vi "Hatch4barCollisionAvoidance.vi"(10 "Current4barSetpoint":dbl, 11 "Hatch Setpoint":dbl) -> (3 "Modified 4bar setpoint":dbl)   [LabVIEW 2018]
uses:
  Infrastructure/Constants.vi
  Robot Global Data.vi
panel:
  out "On floor":bool
  out "currently in bad zone":bool
  out "INtending to move throug floor":bool
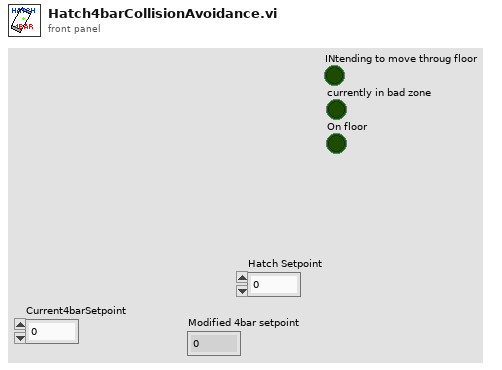
[diagram p1: front panel]
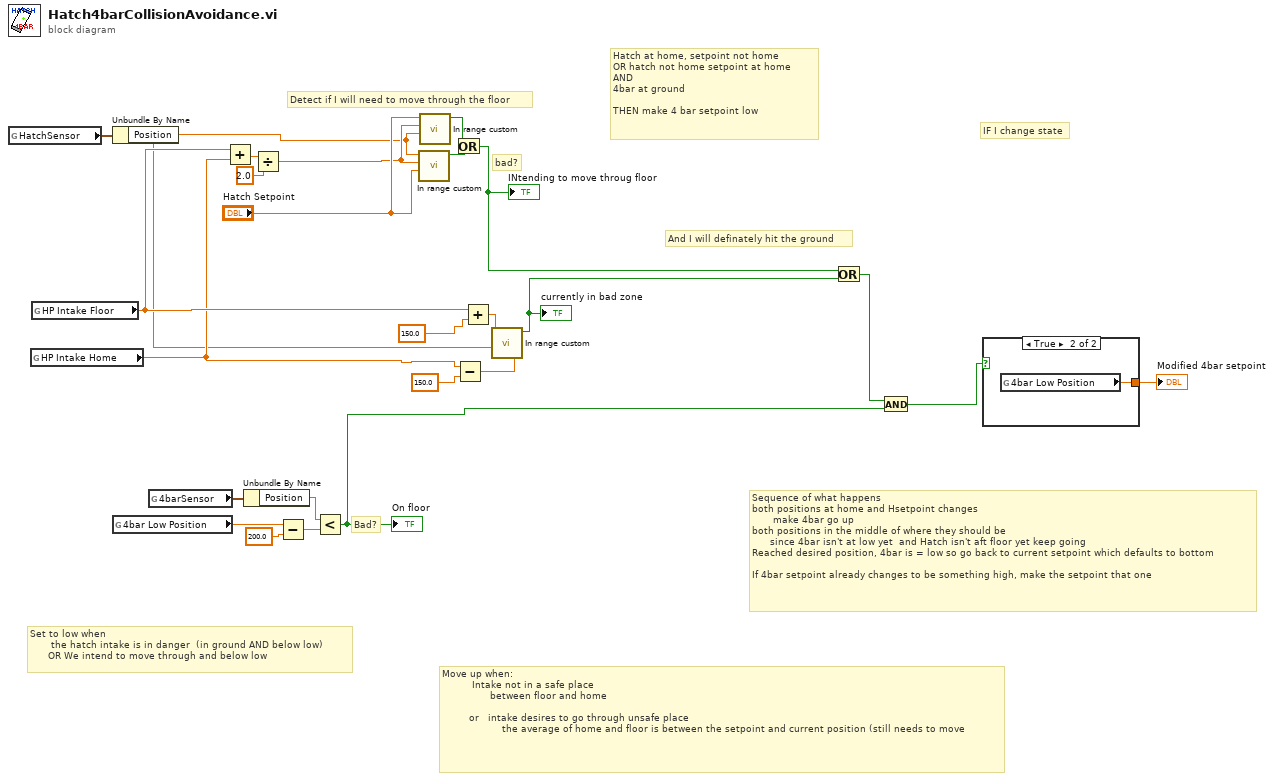
[diagram p0: block diagram]
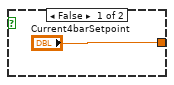
[diagram p2: hidden frame]
diagram:
  # "Set to low when \n       the hatch intake is in danger  (in ground AND below low)\n      OR We intend to move through and below low"
  # "Move up when: \n          Intake not in a safe place\n                between floor and home\n\n         or   intake desires to go through unsafe place\n                    the average of home and floor is between the setpoint and current position (still needs to move"
  # "bad?"
  # "Bad?"
  # "Detect if I will need to move through the floor"
  # "And I will definately hit the ground"
  # "IF I change state"
  # "Sequence of what happens\nboth positions at home and Hsetpoint changes\n       make 4bar go up\nboth positions in the middle of where they should be\n      since 4bar isn't at low yet  and Hatch isn't aft floor yet keep going\nReached desired position, 4bar is = low so go back to current setpoint which defaults to bottom\n\nIf 4bar setpoint already changes to be something high, make the setpoint that one"
  # "Hatch at home, setpoint not home\nOR hatch not home setpoint at home \nAND\n4bar at ground\n\nTHEN make 4 bar setpoint low"
  n1 = global read "Robot Global Data.vi" "HatchSensor"() -> (w25:cluster{"Position":dbl, "Velocity":dbl})
  n2 = global read "Constants.vi" "HP Intake Home"() -> (w10:dbl)
  n3 = global read "Constants.vi" "HP Intake Floor"() -> (w11:dbl)
  n4 = Unbundle By Name(w25) -> ("Position"=w1:dbl)
  n5 = global read "Constants.vi" "4bar Low Position"() -> (w14:dbl)
  n6 = global read "Robot Global Data.vi" "4barSensor"() -> (w24:cluster{"Position":dbl, "Velocity":dbl})
  n7 = Add(x=w11, y=w10) -> (x+y=w21:dbl)
  n8 = Unbundle By Name(w24) -> ("Position"=w22:dbl)
  n9 = Divide(x=w21, y=2.0) -> (x/y=w2:dbl)
  n10 = Subtract(x=w14, y=200.0 ("x")) -> (x-y=w15:dbl)
  n11 = Less?(x=w22, y=w15) -> (x < y?=w17:bool)
  "On floor" <- w17
  n12 = call "In range custom.vi"("Lower limit"="Hatch Setpoint", "x"=w2, "Upper limit"=w1) -> ("In range?"=w5:bool)  [unwired: 8 in]
  n13 = call "In range custom.vi"("Lower limit"=w1, "x"=w2, "Upper limit"="Hatch Setpoint") -> ("In range?"=w4:bool)  [unwired: 8 in]
  n14 = Or(x=w4, y=w5) -> (x .or. y?=w19:bool)
  "INtending to move throug floor" <- w19
  n15 = Subtract(x=w10, y=150.0 ("x")) -> (x-y=w7:dbl)
  n16 = Add(x=w11, y=150.0 ("x")) -> (x+y=w8:dbl)
  n17 = call "In range custom.vi"("Lower limit"=w1, "x"=w7, "Upper limit"=w8) -> ("In range?"=w6:bool)  [unwired: 8 in]
  "currently in bad zone" <- w6
  n18 = Or(x=w19, y=w6) -> (x .or. y?=w18:bool)
  n19 = And(x=w18, y=w17) -> (x .and. y?=w16:bool)
  n20 = case shown="True" w16 {
    tunnel: ["Current4barSetpoint" w27] -> w23
    frame False {
    }
    frame True {
      n21 = global read "Constants.vi" "4bar Low Position"() -> (w27:dbl)
    }
  }
  "Modified 4bar setpoint" <- w23
